vi "MPX Set Path.vi"(4 "stat ref":refnum<vi>, 6 "stop ref":refnum<vi>, 7 "allow wait (True)":bool=TRUE, 8 "error in":errorcluster, 10 "path":string, 11 "session in":T1={"niScope"={"channel cfg"=[], "sessions"=[], "multi cards"=FALSE, "channels"=0, "type"=enum."n/a", "memory [B/chn]"=0, "ext. clock [Hz]"=0.0, "samples count"=0, "use streaming"=FALSE, "proc setup"={"packet size [smpl]"=0, "current timeout [s]"=0.0, "blk2blk timeout [s]"=0.0, "event time"=timestamp(0 s since 1904-01-01), "temp sampl T [s]"=0.0, "data queue"=refnum, "stop notifier"=refnum, "proc ref"=refnum}, "sample width [B]"=0, "ranges [V]"=[], "trigger setup"={"coupling"=1, "level [V]"=0.0, "slope"=0, "mode"=enum."Immediate"}, "fs [Hz]"=0.0, "bitres [bit]"=0, "clock source"=enum."VAL_NO_SOURCE"}, "3458A"={"channels"=[], "sync unit"={"VISA"="", "type"=enum."Picotest U6200A"}, "awg unit"={"type"=enum."Agilent 331xxA to 332xxA", "VISA"="", "enable 10MHz ref"=FALSE, "cmi ckd2"={"VISA"="", "clock source"=enum."Auto", "manual ref clk"=FALSE, "ref clock [Hz]"=0.0}}, "sync mode"=enum."MASTER-SLAVE, MASTER clocked by TIMER", "streaming mode"=FALSE, "idn mode"=enum."Auto", "sampling mode"=enum."DCV", "Ts [s]"=0.0, "sample memory [B]"=0, "proc setup"={"channel id"=0, "packet size [smpl]"=0, "current timeout [s]"=0.0, "blk2blk timeout [s]"=0.0, "event time"=timestamp(0 s since 1904-01-01), "stop notifier"=refnum, "data queues"=[], "proc refs"=[], "bus semaphore"=refnum}, "sample size [B]"=0, "sample count"=0, "aux data"={"channel id"=0, "valid?"=[], "gain [V]"=[], "timestamp [s]"=[], "Ts [s]"=0.0, "abs timestamp"=timestamp(0 s since 1904-01-01), "t [deg C]"=[], "multiplex timestamp [s]"=-1.0, "only multiplex?"=FALSE, "multiplex smpl offset"=0, "overflow?"=FALSE}, "ranges [V]"=[], "aperture [s]"=0.0, "LEVEL trigger"={"edge"=enum."POS", "level [V]"=0.0, "coupling"=enum."DC"}, "trigger mode"=enum."AUTO", "measure temp.?"=FALSE, "disp mesages"=[], "shared bus?"=FALSE, "disable display?"=FALSE, "aper mode"=enum."Manual", "aper rules"=[], "multiplex"={"cycles"=0, "delay [s]"=0.0, "enabled"=FALSE, "overhead [s]"=1.0, "tot smpls"=0, "sub-rec"=0, "overhead [%]"=0.0}, "F8588 lpf"=enum."Off", "F8588 pll"=enum."Off", "F8588 couple"=enum."DC, auto"}, "dsdll"={"dsdll"={"dsdll path"=path "", "dsdll handle"=[], "output devices"=[], "capture devices"=[]}, "channels"=0, "device id"=0, "channel idns"=[], "proc setup"={"packet size [smpl]"=0, "current timeout [s]"=0.0, "blk2blk timeout [s]"=0.0, "event time"=timestamp(0 s since 1904-01-01), "data queue"=refnum, "stop notifier"=refnum, "proc ref"=refnum}, "samples count"=0, "fs [Hz]"=0.0}, "type"=enum."niScope", "channel idn str"=[], "aux instr idn str"=[], "modified?"=FALSE, "simadc"={"channels"=[], "range [V]"=0.0, "Ts step [s]"=0.0, "time [s]"=0.0, "fs [Hz]"=0.0, "count"=0, "smpl offset"=0, "set count"=0, "bit res"=0}, "force rst?"=FALSE, "exit mode"=enum."Immediate reset", "exit dly"=0.0, "exit tmr"=timestamp(0 s since 1904-01-01), "busy?"=FALSE, "accessed?"=FALSE, "multiplex"={"Type"=enum."Dummy", "gen com ssn"={"visa"="", "primary"=enum."None", "secondary"=enum."None", "channels"=[]}, "delay before [s]"=0.0, "delay post [s]"=0.0, "sequence"=[], "enabled"=FALSE, "ref timestamp [s]"=0.0, "idn string"="", "dev niScope"="", "niScope idx"=0}, "keysight dso"={"VISA"="", "channels"=[], "bw limit [Hz]"=0.0, "resolution"=enum."Auto", "trig noise reject"=enum."Normal", "N"=0, "trigger config"={"trigger source"=enum."Immediate", "level [V]"=0.0, "trigger slope"=enum."Negative"}, "fs [Hz]"=0.0, "timeout stop"=timestamp(0 s since 1904-01-01), "waiting for opc"=FALSE, "fetch offset [smpl]"=0, "abs timestamp"=timestamp(0 s since 1904-01-01), "ranges [V]"=[]}, "cdaq"={"mclk [Hz]"=12800000.0, "ADC task"="", "mclk reference"="", "fs [Hz]"=50000.0, "queue adc cmd"=refnum, "queue adc data"=refnum, "adc proc ref"=refnum, "channels"=[], "last channels"=[], "timeout"=timestamp(0 s since 1904-01-01), "N"=1000}} {"cdaq"."last channels"."Channel id" min=0 step=1; "cdaq"."channels"."Channel id" min=0 step=1; "keysight dso"."bw limit [Hz]" format="%#_6p"; "keysight dso"."channels"."Offset [V]" min=0.0 format="%#_6p"; "keysight dso"."channels"."Range [Vpk]" min=0.0 format="%#_6p"; "keysight dso"."channels"."Channel" min=1; "3458A"."channels"."Range [Vpk]" min=0.0; "niScope"."trigger setup"."level [V]" format="%.2f"; "niScope"."trigger setup"."coupling" items=["AC"=0, "DC"=1, "HF Reject"=3, "LF Reject"=4, "AC Plus HF Reject"=1001]; "niScope"."channel cfg"."Range [Vpk]" min=0.0; "niScope"."channel cfg"."Channel" min=0}) -> (0 "error out":errorcluster, 3 "session out":T1={"niScope"={"channel cfg"=[], "sessions"=[], "multi cards"=FALSE, "channels"=0, "type"=enum."n/a", "memory [B/chn]"=0, "ext. clock [Hz]"=0.0, "samples count"=0, "use streaming"=FALSE, "proc setup"={"packet size [smpl]"=0, "current timeout [s]"=0.0, "blk2blk timeout [s]"=0.0, "event time"=timestamp(0 s since 1904-01-01), "temp sampl T [s]"=0.0, "data queue"=refnum, "stop notifier"=refnum, "proc ref"=refnum}, "sample width [B]"=0, "ranges [V]"=[], "trigger setup"={"coupling"=1, "level [V]"=0.0, "slope"=0, "mode"=enum."Immediate"}, "fs [Hz]"=0.0, "bitres [bit]"=0, "clock source"=enum."VAL_NO_SOURCE"}, "3458A"={"channels"=[], "sync unit"={"VISA"="", "type"=enum."Picotest U6200A"}, "awg unit"={"type"=enum."Agilent 331xxA to 332xxA", "VISA"="", "enable 10MHz ref"=FALSE, "cmi ckd2"={"VISA"="", "clock source"=enum."Auto", "manual ref clk"=FALSE, "ref clock [Hz]"=0.0}}, "sync mode"=enum."MASTER-SLAVE, MASTER clocked by TIMER", "streaming mode"=FALSE, "idn mode"=enum."Auto", "sampling mode"=enum."DCV", "Ts [s]"=0.0, "sample memory [B]"=0, "proc setup"={"channel id"=0, "packet size [smpl]"=0, "current timeout [s]"=0.0, "blk2blk timeout [s]"=0.0, "event time"=timestamp(0 s since 1904-01-01), "stop notifier"=refnum, "data queues"=[], "proc refs"=[], "bus semaphore"=refnum}, "sample size [B]"=0, "sample count"=0, "aux data"={"channel id"=0, "valid?"=[], "gain [V]"=[], "timestamp [s]"=[], "Ts [s]"=0.0, "abs timestamp"=timestamp(0 s since 1904-01-01), "t [deg C]"=[], "multiplex timestamp [s]"=-1.0, "only multiplex?"=FALSE, "multiplex smpl offset"=0, "overflow?"=FALSE}, "ranges [V]"=[], "aperture [s]"=0.0, "LEVEL trigger"={"edge"=enum."POS", "level [V]"=0.0, "coupling"=enum."DC"}, "trigger mode"=enum."AUTO", "measure temp.?"=FALSE, "disp mesages"=[], "shared bus?"=FALSE, "disable display?"=FALSE, "aper mode"=enum."Manual", "aper rules"=[], "multiplex"={"cycles"=0, "delay [s]"=0.0, "enabled"=FALSE, "overhead [s]"=1.0, "tot smpls"=0, "sub-rec"=0, "overhead [%]"=0.0}, "F8588 lpf"=enum."Off", "F8588 pll"=enum."Off", "F8588 couple"=enum."DC, auto"}, "dsdll"={"dsdll"={"dsdll path"=path "", "dsdll handle"=[], "output devices"=[], "capture devices"=[]}, "channels"=0, "device id"=0, "channel idns"=[], "proc setup"={"packet size [smpl]"=0, "current timeout [s]"=0.0, "blk2blk timeout [s]"=0.0, "event time"=timestamp(0 s since 1904-01-01), "data queue"=refnum, "stop notifier"=refnum, "proc ref"=refnum}, "samples count"=0, "fs [Hz]"=0.0}, "type"=enum."niScope", "channel idn str"=[], "aux instr idn str"=[], "modified?"=FALSE, "simadc"={"channels"=[], "range [V]"=0.0, "Ts step [s]"=0.0, "time [s]"=0.0, "fs [Hz]"=0.0, "count"=0, "smpl offset"=0, "set count"=0, "bit res"=0}, "force rst?"=FALSE, "exit mode"=enum."Immediate reset", "exit dly"=0.0, "exit tmr"=timestamp(0 s since 1904-01-01), "busy?"=FALSE, "accessed?"=FALSE, "multiplex"={"Type"=enum."Dummy", "gen com ssn"={"visa"="", "primary"=enum."None", "secondary"=enum."None", "channels"=[]}, "delay before [s]"=0.0, "delay post [s]"=0.0, "sequence"=[], "enabled"=FALSE, "ref timestamp [s]"=0.0, "idn string"="", "dev niScope"="", "niScope idx"=0}, "keysight dso"={"VISA"="", "channels"=[], "bw limit [Hz]"=0.0, "resolution"=enum."Auto", "trig noise reject"=enum."Normal", "N"=0, "trigger config"={"trigger source"=enum."Immediate", "level [V]"=0.0, "trigger slope"=enum."Negative"}, "fs [Hz]"=0.0, "timeout stop"=timestamp(0 s since 1904-01-01), "waiting for opc"=FALSE, "fetch offset [smpl]"=0, "abs timestamp"=timestamp(0 s since 1904-01-01), "ranges [V]"=[]}, "cdaq"={"mclk [Hz]"=12800000.0, "ADC task"="", "mclk reference"="", "fs [Hz]"=50000.0, "queue adc cmd"=refnum, "queue adc data"=refnum, "adc proc ref"=refnum, "channels"=[], "last channels"=[], "timeout"=timestamp(0 s since 1904-01-01), "N"=1000}} {"cdaq"."last channels"."Channel id" min=0 step=1; "cdaq"."channels"."Channel id" min=0 step=1; "keysight dso"."bw limit [Hz]" format="%#_6p"; "keysight dso"."channels"."Offset [V]" min=0.0 format="%#_6p"; "keysight dso"."channels"."Range [Vpk]" min=0.0 format="%#_6p"; "keysight dso"."channels"."Channel" min=1; "3458A"."channels"."Range [Vpk]" min=0.0; "niScope"."trigger setup"."level [V]" format="%.2f"; "niScope"."trigger setup"."coupling" items=["AC"=0, "DC"=1, "HF Reject"=3, "LF Reject"=4, "AC Plus HF Reject"=1001]; "niScope"."channel cfg"."Range [Vpk]" min=0.0; "niScope"."channel cfg"."Channel" min=0})   [LabVIEW 2013]
doc: "Sets path of the multiplexer device. Applies pre and post delay.\nStop ref and Stat ref can be used to print delay status to a string indicator and to stop delay by stop boolean."
uses:
  ADC Session.ctl
  drivers/niScope/niScope Session.ctl
  drivers/niScope/niScope Virtual Channel Config.ctl
  drivers/niScope/niScope Virtual Channel Mode.ctl
  drivers/niScope/niScope Virtual Channel Input Z.ctl
  drivers/niScope/niScope Virtual Channel Coupling.ctl
  drivers/niScope/niScope Type.ctl
  drivers/niScope/niScope Digitizing Process Options.ctl
  drivers/niScope/niScope Data Packet.ctl
  drivers/niScope/niScope Trigger Setup.ctl
  <instrlib>/niScope/Controls/niScope trigger coupling.ctl
  <instrlib>/niScope/Controls/niScope trigger slope.ctl
  drivers/niScope/niScope Reference Clock.ctl
  drivers/DMM/3458A Digitizer Session.ctl
  drivers/DMM/3458A Virtual Channel Config.ctl
  drivers/Counter/Counter Session.ctl
  drivers/Counter/Counter Type.ctl
  drivers/AWG/AWG Session.ctl
  drivers/AWG/AWG Type.ctl
  drivers/AWG/CMI Clock Divider v2/CMI ckd2 Session.ctl
  drivers/AWG/CMI Clock Divider v2/CMI ckd2 Source Mode.ctl
  drivers/DMM/3458A Sync Mode.ctl
  drivers/DMM/3458A Idn Mode.ctl
  drivers/DMM/3458A Digitizing Low Levels/Configure/Sampling Mode.ctl
  drivers/DMM/3458A Digitizing Process Options.ctl
  drivers/DMM/3458A Data Packet.ctl
  drivers/DMM/3458A Aux Record Data.ctl
  drivers/DMM/3458A Digitizing Low Levels/Configure/Level Setup.ctl
  drivers/DMM/3458A Digitizing Low Levels/Configure/First Sample Trigger.ctl
  drivers/DMM/3458A Aperture Selection Mode.ctl
  drivers/DMM/3458A Multiplexing Config.ctl
  drivers/Fluke 8588A/F8588A Low Pass Filter.ctl
  drivers/Fluke 8588A/F8588A Phase Lock.ctl
  drivers/Fluke 8588A/F8588A Coupling.ctl
  drivers/dsdll/DSDLL Session.ctl
  drivers/dsdll/dsdll.lvlibp/dsdll_instance.ctl
  drivers/dsdll/dsdll.lvlibp/dsdll_device_record.ctl
  drivers/dsdll/DSDLL Process Config.ctl
  drivers/dsdll/DSDLL Data Packet.ctl
  ADC Type.ctl
  drivers/simulated_adc/SimAdc Config.ctl
  drivers/simulated_adc/SimAdc Channel Cfg.ctl
  ADC On Close Action.ctl
  MPX Session.ctl
  MPX Type.ctl
  drivers/Multiplexers/Generic COM/GCOMM Session.ctl
  drivers/Multiplexers/Generic COM/GCOMM Signal.ctl
  drivers/Multiplexers/Generic COM/GCOMM Virtual Channel.ctl
  drivers/Multiplexers/Generic COM/GCOMM Logic State.ctl
  drivers/Agilent DSO 90000/Virtual Digitizer/KeDSO session.ctl
  drivers/Agilent DSO 90000/Virtual Digitizer/KeDSO Virtual Channel.ctl
  drivers/Agilent DSO 90000/Virtual Digitizer/KeDSO Trigger Setup.ctl
  drivers/Agilent DSO 90000/Virtual Digitizer/KeDSO Trigger Source.ctl
  drivers/cdaq/cDAQ Session.ctl
  drivers/cdaq/low_level_old/cdaq_anal_adc_command.ctl
  drivers/cdaq/low_level_old/cdaq_anal_adc_data.ctl
  drivers/cdaq/cDAQ Virtual Channel.ctl
  varilib/varilib.lvlib
  <vilib>/Utility/error.llb/Error Cluster From Error Code.vi
  <vilib>/ErrorRing/Error Ring.xnode
  drivers/niScope/niScope Virtual Digitizer.lvlib
  drivers/DMM/3458A Virtual Digitizer.lvlib
  drivers/Counter/Counter.lvlib
  drivers/AWG/AWG.lvlib
  drivers/DMM/3458A Digitizing Low Levels/3458A Digitizing Low Levels.lvlib
  drivers/dsdll/dsdll.lvlibp
  drivers/dsdll/DSDLL Virtual Digitizer.lvlib
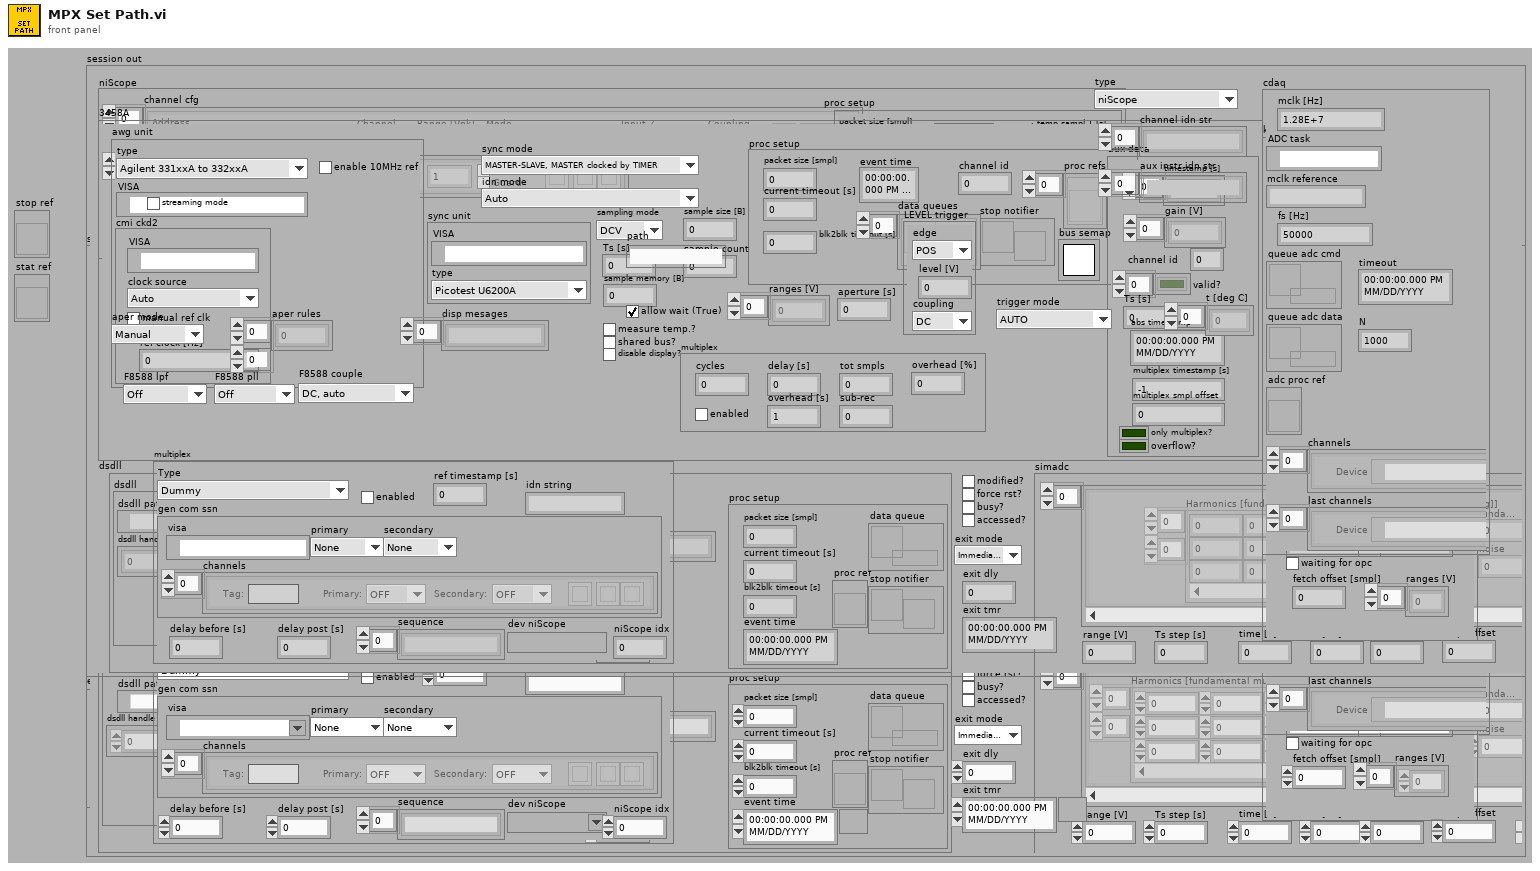
[diagram p1: front panel]
types:
  T1 = typedef "ADC Session.ctl" = cluster{"niScope":T2, "3458A":T13, "dsdll":T34, "type":T38, "channel idn str":string[], "aux instr idn str":string[], "modified?":bool, "simadc":T39, "force rst?":bool, "exit mode":T41, "exit dly":dbl, "exit tmr":timestamp, "busy?":bool, "accessed?":bool, "multiplex":T42, "keysight dso":T48, "cdaq":T52}
  T2 = typedef "niScope Virtual Digitizer.lvlib/niScope Session.ctl" = cluster{"channel cfg":T3[], "sessions":refnum<k20>[], "multi cards":bool, "channels":i32, "type":T7, "memory [B/chn]":i32, "ext. clock [Hz]":dbl, "samples count":i64, "use streaming":bool, "proc setup":T8, "sample width [B]":i32, "ranges [V]":dbl[], "trigger setup":T9, "fs [Hz]":dbl, "bitres [bit]":i32, "clock source":T12}
  T3 = typedef "niScope Virtual Digitizer.lvlib/niScope Virtual Channel Config.ctl" = cluster{"Address":refnum<k15>, "Channel":i32, "Mode":T4, "Input Z":T5, "Coupling":T6, "Range [Vpk]":dbl, "btn clr":bool, "btn up":bool, "btn down":bool}
  T4 = typedef "niScope Virtual Digitizer.lvlib/niScope Virtual Channel Mode.ctl" = enum16{"Single ended", "Unbal. differential", "Differential"}
  T5 = typedef "niScope Virtual Digitizer.lvlib/niScope Virtual Channel Input Z.ctl" = enum16{"1 MOhm", "50 Ohm"}
  T6 = typedef "niScope Virtual Digitizer.lvlib/niScope Virtual Channel Coupling.ctl" = enum16{"AC", "DC", "GND"}
  T7 = typedef "niScope Virtual Digitizer.lvlib/niScope Type.ctl" = enum16{"n/a", "5922"}
  T8 = typedef "niScope Virtual Digitizer.lvlib/niScope Digitizing Process Options.ctl" = cluster{"packet size [smpl]":i64, "current timeout [s]":dbl, "blk2blk timeout [s]":dbl, "event time":timestamp, "temp sampl T [s]":dbl, "data queue":refnum<queue>, "stop notifier":refnum<notifier>, "proc ref":refnum<vi>}
  T9 = typedef "niScope Virtual Digitizer.lvlib/niScope Trigger Setup.ctl" = cluster{"coupling":T10, "level [V]":dbl, "slope":T11, "mode":enum16{"Immediate", "External", "Level"}}
  T10 = typedef "niScope trigger coupling.ctl" = u16
  T11 = typedef "niScope trigger slope.ctl" = i32
  T12 = typedef "niScope Virtual Digitizer.lvlib/niScope Reference Clock.ctl" = enum16{"VAL_NO_SOURCE", "VAL_CLK_IN", "VAL_PXI_CLOCK", "VAL_EXTERNAL"}
  T13 = typedef "3458A Virtual Digitizer.lvlib/3458A Digitizer Session.ctl" = cluster{"channels":T14[], "sync unit":T15, "awg unit":T17, "sync mode":T21, "streaming mode":bool, "idn mode":T22, "sampling mode":T23, "Ts [s]":dbl, "sample memory [B]":i32, "proc setup":T24, "sample size [B]":i32, "sample count":i32, "aux data":T26, "ranges [V]":dbl[], "aperture [s]":dbl, "LEVEL trigger":T27, "trigger mode":T28, "measure temp.?":bool, "disp mesages":string[], "shared bus?":bool, "disable display?":bool, "aper mode":T29, "aper rules":dbl[][], "multiplex":T30, "F8588 lpf":T31, "F8588 pll":T32, "F8588 couple":T33}
  T14 = typedef "3458A Virtual Digitizer.lvlib/3458A Virtual Channel Config.ctl" = cluster{"VISA":refnum<visa-resource-name>, "Range [Vpk]":dbl, "btn clr":bool, "btn up":bool, "btn down":bool, "F8588":bool, "F8588 guard":bool}
  T15 = typedef "Counter.lvlib/Counter Session.ctl" = cluster{"VISA":refnum<visa-resource-name>, "type":T16}
  T16 = typedef "Counter.lvlib/Counter Type.ctl" = enum16{"Picotest U6200A", "dummy"}
  T17 = typedef "AWG.lvlib/AWG Session.ctl" = cluster{"type":T18, "VISA":refnum<visa-resource-name>, "enable 10MHz ref":bool, "cmi ckd2":T19}
  T18 = typedef "AWG.lvlib/AWG Type.ctl" = enum16{"Agilent 331xxA to 332xxA", "Agilent 335xxA to 336xxA", "Tektronix AFG3101C", "CMI Clock Divider v2", "dummy"}
  T19 = typedef "AWG.lvlib/CMI ckd2 Session.ctl" = cluster{"VISA":refnum<visa-resource-name>, "clock source":T20, "manual ref clk":bool, "ref clock [Hz]":dbl}
  T20 = typedef "AWG.lvlib/CMI ckd2 Source Mode.ctl" = enum16{"Auto", "LF clock", "HF clock", "Internal"}
  T21 = typedef "3458A Virtual Digitizer.lvlib/3458A Sync Mode.ctl" = enum16{"MASTER-SLAVE, MASTER clocked by TIMER", "MASTER-SLAVE, MASTER clocked by AWG", "ALL clocked by AWG", "MASTER-SLAVE, ALL clocked by TIMER", "ALL clocked by AWG with DFLL"}
  T22 = typedef "3458A Virtual Digitizer.lvlib/3458A Idn Mode.ctl" = enum16{"Auto", "Sequential (chn A, chn B, ...)", "From calibration string"}
  T23 = typedef "3458A Virtual Digitizer.lvlib/3458A Digitizing Low Levels.lvlib/Sampling Mode.ctl" = enum16{"DCV", "DSDC", "DSAC"}
  T24 = typedef "3458A Virtual Digitizer.lvlib/3458A Digitizing Process Options.ctl" = cluster{"channel id":i32, "packet size [smpl]":i32, "current timeout [s]":dbl, "blk2blk timeout [s]":dbl, "event time":timestamp, "stop notifier":refnum<notifier>, "data queues":refnum<queue>[], "proc refs":refnum<vi>[], "bus semaphore":T25}
  T25 = typedef "Semaphore RefNum" = refnum<k1>
  T26 = typedef "3458A Virtual Digitizer.lvlib/3458A Aux Record Data.ctl" = cluster{"channel id":i32, "valid?":bool[], "gain [V]":dbl[], "timestamp [s]":dbl[], "Ts [s]":dbl, "abs timestamp":timestamp, "t [deg C]":dbl[], "multiplex timestamp [s]":dbl, "only multiplex?":bool, "multiplex smpl offset":i64, "overflow?":bool}
  T27 = typedef "3458A Virtual Digitizer.lvlib/3458A Digitizing Low Levels.lvlib/Level Setup.ctl" = cluster{"edge":enum16{"POS", "NEG"}, "level [V]":dbl, "coupling":enum16{"DC", "AC"}}
  T28 = typedef "3458A Virtual Digitizer.lvlib/3458A Digitizing Low Levels.lvlib/First Sample Trigger.ctl" = enum16{"AUTO", "EXT", "SYN", "SGL", "HOLD", "LEVEL"}
  T29 = typedef "3458A Virtual Digitizer.lvlib/3458A Aperture Selection Mode.ctl" = enum16{"Manual", "Maximum", "Table"}
  T30 = typedef "3458A Multiplexing Config.ctl" = cluster{"cycles":i32, "delay [s]":dbl, "enabled":bool, "overhead [s]":dbl, "tot smpls":i64, "sub-rec":i32, "overhead [%]":dbl}
  T31 = typedef "F8588A Low Pass Filter.ctl" = enum16{"Off", "100 kHz", "3 MHz"}
  T32 = typedef "F8588A Phase Lock.ctl" = enum16{"Off", "1 MHz", "10 MHz"}
  T33 = typedef "F8588A Coupling.ctl" = enum16{"AC, 1 MOhm", "AC, 10 MOhm", "DC, 1 MOhm", "DC, 10 MOhm", "DC, auto"}
  T34 = typedef "DSDLL Virtual Digitizer.lvlib/DSDLL Session.ctl" = cluster{"dsdll":T35, "channels":i32, "device id":i32, "channel idns":string[], "proc setup":T37, "samples count":i32, "fs [Hz]":dbl}
  T35 = typedef "dsdll.lvlibp/dsdll_instance.ctl" = cluster{"dsdll path":path, "dsdll handle":u8[], "output devices":T36[], "capture devices":T36[]}
  T36 = typedef "dsdll.lvlibp/dsdll_device_record.ctl" = cluster{"guid":u8[], "name":string}
  T37 = typedef "DSDLL Virtual Digitizer.lvlib/DSDLL Process Config.ctl" = cluster{"packet size [smpl]":i32, "current timeout [s]":dbl, "blk2blk timeout [s]":dbl, "event time":timestamp, "data queue":refnum<queue>, "stop notifier":refnum<notifier>, "proc ref":refnum<vi>}
  T38 = typedef "ADC Type.ctl" = enum16{"niScope", "3458A", "DirectSound DLL", "Keysight DSO", "cDAQ ADC", "dummy"}
  T39 = typedef "SimAdc Config.ctl" = cluster{"channels":T40[], "range [V]":dbl, "Ts step [s]":dbl, "time [s]":dbl, "fs [Hz]":dbl, "count":i64, "smpl offset":i64, "set count":i64, "bit res":i32}
  T40 = typedef "SimAdc Channel Cfg.ctl" = cluster{"harmonics":dbl[][], "btn clear":bool, "noise":dbl, "fundamental [Hz]":dbl}
  T41 = typedef "ADC On Close Action.ctl" = enum16{"Immediate reset", "Delayed reset"}
  T42 = typedef "MPX Session.ctl" = cluster{"Type":T43, "gen com ssn":T44, "delay before [s]":dbl, "delay post [s]":dbl, "sequence":string[], "enabled":bool, "ref timestamp [s]":dbl, "idn string":string, "dev niScope":refnum<k15>, "niScope idx":i32}
  T43 = typedef "MPX Type.ctl" = enum16{"Dummy", "Generic - COM port", "Generic - niScope PFI"}
  T44 = typedef "GCOMM Session.ctl" = cluster{"visa":refnum<visa-resource-name>, "primary":T45, "secondary":T45, "channels":T46[]}
  T45 = typedef "GCOMM Signal.ctl" = enum16{"None", "DTR", "RTS"}
  T46 = typedef "GCOMM Virtual Channel.ctl" = cluster{"Primary:":T47, "Secondary:":T47, "btn clr":bool, "btn up":bool, "btn down":bool, "Tag:":string}
  T47 = typedef "GCOMM Logic State.ctl" = enum16{"OFF", "ON"}
  T48 = typedef "KeDSO session.ctl" = cluster{"VISA":refnum<visa-resource-name>, "channels":T49[], "bw limit [Hz]":dbl, "resolution":enum16{"Auto", "Bits 9", "Bits 10", "Bits 11", "Bits 12"}, "trig noise reject":enum16{"Normal", "High Sensitivity"}, "N":i64, "trigger config":T50, "fs [Hz]":dbl, "timeout stop":timestamp, "waiting for opc":bool, "fetch offset [smpl]":i64, "abs timestamp":timestamp, "ranges [V]":dbl[]}
  T49 = typedef "KeDSO Virtual Channel.ctl" = cluster{"Channel":i32, "Range [Vpk]":dbl, "btn clr":bool, "btn up":bool, "btn down":bool, "Offset [V]":dbl, "Coupling":enum16{"DC", "DC50", "AC", "LFR1"}, "bw limit enab":bool}
  T50 = typedef "KeDSO Trigger Setup.ctl" = cluster{"trigger source":T51, "level [V]":dbl, "trigger slope":enum16{"Negative", "Positive", "Either"}}
  T51 = typedef "KeDSO Trigger Source.ctl" = enum16{"Immediate", "Level", "AUX"}
  T52 = typedef "cDAQ Session.ctl" = cluster{"mclk [Hz]":dbl, "ADC task":refnum<k21>, "mclk reference":string, "fs [Hz]":dbl, "queue adc cmd":refnum<queue>, "queue adc data":refnum<queue>, "adc proc ref":refnum<vi>, "channels":T53[], "last channels":T53[], "timeout":timestamp, "N":i32}
  T53 = typedef "cDAQ Virtual Channel.ctl" = cluster{"Device":tag, "Channel id":i32, "btn clr":bool, "btn up":bool, "btn down":bool}
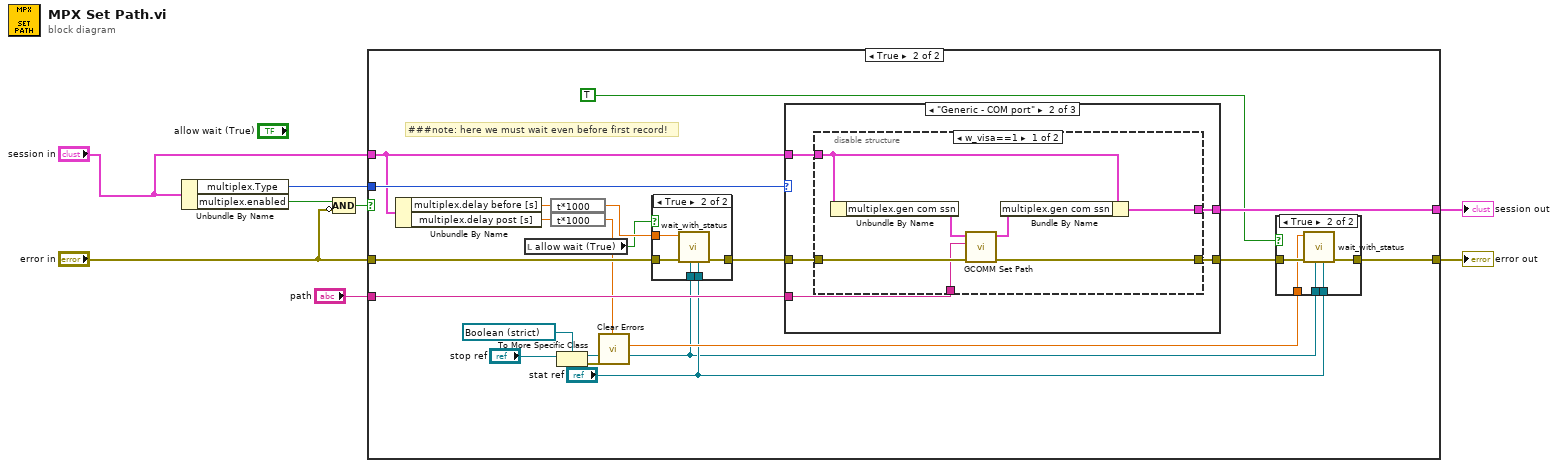
[diagram p0: block diagram]
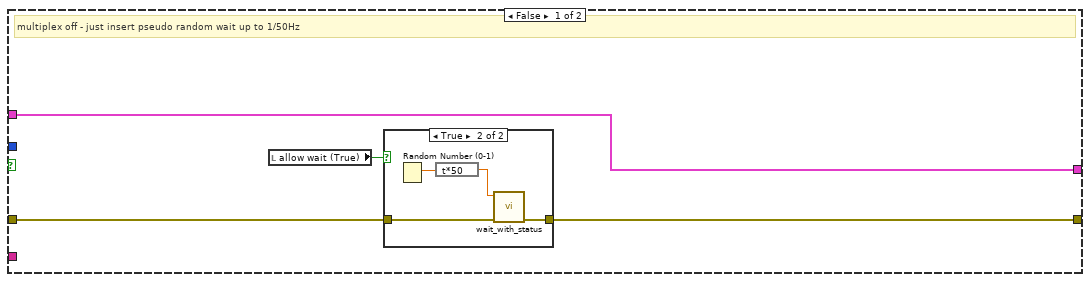
[diagram p2: hidden frame]
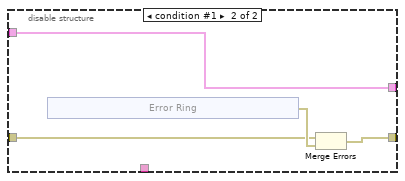
[diagram p7: hidden frame]
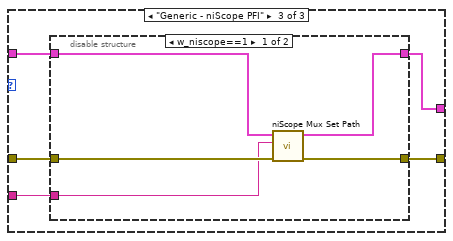
[diagram p8: hidden frame]
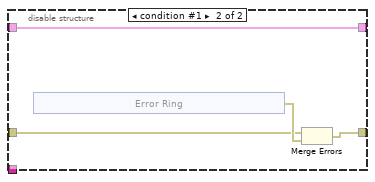
[diagram p9: hidden frame]
diagram:
  n1 = Unbundle By Name("session in") -> ("multiplex.Type"=w6:T43, "multiplex.enabled"=w8:bool)
  n2 = Compound Arithmetic op=AND(w8, invert "error in") -> (w7:bool)
  n3 = case shown="True" w7 {
    tunnel: w6 -> [_ w36]
    tunnel: "error in" -> [w11 w32]
    tunnel: "session in" -> [w12 w33]
    tunnel: [w12 w35] -> w5
    tunnel: [w10 w27] -> w4
    tunnel: "path" -> [_ w34]
    frame False {
      # "multiplex off - just insert pseudo random wait up to 1/50Hz"
      n4 = local read "allow wait (True)"() -> (w9:bool)
      n5 = case shown="True" w9 {
        tunnel: w11 -> [w13 w17]
        tunnel: [w13 w16] -> w10
        frame False {
        }
        frame True {
          n6 = Random Number (0-1)() -> (number: 0 to 1=w15:dbl)
          n7 = expression code="t*50"(w15) -> (w14:dbl)
          n8 = call "wait_with_status.vi"("error in"=w17, "ms to wait"=w14) -> ("error out"=w16:errorcluster)  [unwired: 9 in]
        }
      }
    }
    frame True {
      # "###note: here we must wait even before first record!"
      n9 = Unbundle By Name(w33) -> ("multiplex.delay before [s]"=w29:dbl, "multiplex.delay post [s]"=w26:dbl)
      n10 = local read "allow wait (True)"() -> (w18:bool)
      n11 = expression code="t*1000"(w29) -> (w30:dbl)
      n12 = expression code="t*1000"(w26) -> (w25:dbl)
      n13 = To More Specific Class(target class=refnum<vi> refnum ("OK Button"), reference="stop ref") -> (specific class reference=w23:refnum<vi>, error out=w20:errorcluster)  [unwired: 1 in]
      n14 = call <vilib>:"Clear Errors.vi"("error in (no error)"=w20) -> ()  [unwired: 6 in, 1 out]
      n15 = case shown="True" w18 {
        tunnel: w32 -> [w43 w48]
        tunnel: [w43 w47] -> w31
        tunnel: w30 -> [_ w46]
        tunnel: "stat ref" -> [_ w45]
        tunnel: w23 -> [_ w44]
        frame False {
        }
        frame True {
          n16 = call "wait_with_status.vi"("stat ref"=w45, "stop ref"=w44, "error in"=w48, "ms to wait"=w46) -> ("error out"=w47:errorcluster)  [unwired: 7 in]
        }
      }
      n17 = case shown="\"Generic - COM port\"" w36 {
        tunnel: w31 -> [w49 w55 w76]
        tunnel: w33 -> [w50 w54 w74]
        tunnel: [w50 w53 w73] -> w35
        tunnel: [w49 w52 w75] -> w28
        tunnel: w34 -> [_ w51 w72]
        frame Default {
        }
        frame "Generic - COM port" {
          n18 = disable-structure shown="w_visa==1" {
            disable-tunnel: w55 -> [w62 w64]
            disable-tunnel: w54 -> [w60 w66]
            disable-tunnel: [w58 w66] -> w53
            disable-tunnel: [w57 w63] -> w52
            disable-tunnel: w51 -> [w56 _]
            frame condition #0 (active) {
              n19 = Unbundle By Name(w60) -> ("multiplex.gen com ssn"=w61:T44)
              n20 = call "GCOMM Set Path.vi"("error in"=w62, "path"=w56, "session in"=w61) -> ("error out"=w57:errorcluster, "session out"=w59:T44)  [unwired: 7 in]
              n21 = Bundle By Name(cluster=w60, "multiplex.gen com ssn"=w59) -> (w58:T1)
            }
            frame condition #1 {
              n22 = xnode "Error Ring"() -> ("error out"=w65:errorcluster)
              n23 = Merge Errors(w64, w65) -> (w63:errorcluster)
            }
          }
        }
        frame "Generic - niScope PFI" {
          n24 = disable-structure shown="w_niscope==1" {
            disable-tunnel: w76 -> [w81 w84]
            disable-tunnel: [w78 w83] -> w75
            disable-tunnel: w74 -> [w80 w82]
            disable-tunnel: [w77 w82] -> w73
            disable-tunnel: w72 -> [w79 _]
            frame condition #0 (active) {
              n25 = call "niScope Mux Set Path.vi"("error in"=w81, "path name ('')"=w79, "adc session in"=w80) -> ("error out"=w78:errorcluster, "adc session out"=w77:T1)  [unwired: 7 in]
            }
            frame condition #1 {
              n26 = xnode "Error Ring"() -> ("error out"=w85:errorcluster)
              n27 = Merge Errors(w84, w85) -> (w83:errorcluster)
            }
          }
        }
      }
      n28 = case shown="True" TRUE {
        tunnel: w28 -> [w37 w42]
        tunnel: [w37 w41] -> w27
        tunnel: w25 -> [_ w40]
        tunnel: "stat ref" -> [_ w39]
        tunnel: w23 -> [_ w38]
        frame False {
        }
        frame True {
          n29 = call "wait_with_status.vi"("stat ref"=w39, "stop ref"=w38, "error in"=w42, "ms to wait"=w40) -> ("error out"=w41:errorcluster)  [unwired: 7 in]
        }
      }
    }
  }
  "error out" <- w4
  "session out" <- w5
